vi "Toggle Selection.vi"(8 "error in (no error)":errorcluster, 10 "Tag":string, 11 "TreeSelectionHierarchal in":refnum<class "TreeSelectionHierarchal.lvclass">) -> (0 "error out":errorcluster, 3 "TreeSelectionHierarchal out":refnum<class "TreeSelectionHierarchal.lvclass">)   [LabVIEW 2015, in "TreeSelectionHierarchal.lvclass"]
doc: "<b> </b> <b> </b>\n©2016 Q Software Innovations, LLC (QSI)\nwritten by Quentin Alldredge\nproduced in LabVIEW 2015\n\nsupport@qsoftwareinnovations.com\nwww.qsoftwareinnovations.com\n\nAll rights reserved.\n\nRedistribution and use in source and binary forms, with or without modification, are permitted provided that the following conditions are met:\n\n * Redistributions of source code must retain the above copyright notice, this list of conditions and the following disclaimer.\n * Redistributions in binary form must reproduce the above copyright notice, this list of conditions and the following disclaimer in the documentation and/or other materials provided with the distribution.\n * Neither the name of Q Software Innovations, LLC. nor the names of its contributors may be used to endorse or promote products derived from this software without specific prior written permission.\n\nTHIS SOFTWARE IS PROVIDED BY THE COPYRIGHT HOLDERS AND CONTRIBUTORS \"AS IS\" AND ANY EXPRESS OR IMPLIED WARRANTIES, INCLUDING, BUT NOT LIMITED TO, THE IMPLIED WARRANTIES OF MERCHANTABILITY AND FITNESS FOR A PARTICULAR PURPOSE ARE DISCLAIMED. IN NO EVENT SHALL THE COPYRIGHT OWNER OR CONTRIBUTORS BE LIABLE FOR ANY DIRECT, INDIRECT, INCIDENTAL, SPECIAL, EXEMPLARY, OR CONSEQUENTIAL DAMAGES (INCLUDING, BUT NOT LIMITED TO, PROCUREMENT OF SUBSTITUTE GOODS OR SERVICES; LOSS OF USE, DATA, OR PROFITS; OR BUSINESS INTERRUPTION) HOWEVER CAUSED AND ON ANY THEORY OF LIABILITY, WHETHER IN CONTRACT, STRICT LIABILITY, OR TORT (INCLUDING NEGLIGENCE OR OTHERWISE) ARISING IN ANY WAY OUT OF THE USE OF THIS SOFTWARE, EVEN IF ADVISED OF THE POSSIBILITY OF SUCH DAMAGE."
uses:
  TreeSelectionHierarchal.lvclass
  TreeControl/TreeControl.lvclass
  TreeSelection/TreeSelection.lvclass
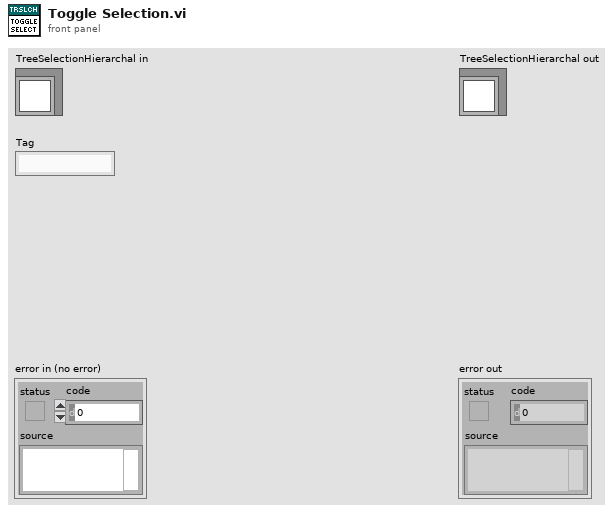
[diagram p1: front panel]
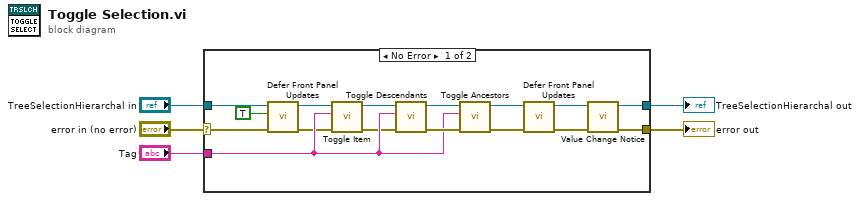
[diagram p0: block diagram]
diagram:
  n1 = case shown="No Error" "error in (no error)" {
    selector: "error in (no error)" -> [w20 w22]
    tunnel: "TreeSelectionHierarchal in" -> [w21 w23]
    tunnel: [w8 w23] -> w3
    tunnel: [w6 w22] -> w2
    tunnel: "Tag" -> [w12 _]
    frame No Error {
      n2 = call "Defer Front Panel Updates.vi"("error in (no error)"=w20, "Defer Panel Updates (F)"=TRUE, "Tree in"=w21) -> ("error out"=w11:errorcluster, "Tree (dup)"=w14:refnum<class "TreeSelectionHierarchal.lvclass">)  [unwired: 7 in]
      n3 = call "Toggle Item.vi"("error in (no error)"=w11, "Tag"=w12, "TreeSelection in"=w14) -> ("error out"=w10:errorcluster, "TreeSelection out"=w13:refnum<class "TreeSelectionHierarchal.lvclass">)  [unwired: 7 in]
      n4 = call "Toggle Descendants.vi"("error in (no error)"=w10, "Tag"=w12, "TreeHier in"=w13) -> ("error out"=w18:errorcluster, "TreeHier out"=w19:refnum<class "TreeSelectionHierarchal.lvclass">)  [unwired: 7 in]
      n5 = call "Toggle Ancestors.vi"("error in (no error)"=w18, "Tag"=w12, "TreeHier in"=w19) -> ("error out"=w15:errorcluster, "TreeHier out"=w16:refnum<class "TreeSelectionHierarchal.lvclass">)  [unwired: 7 in]
      n6 = call "Defer Front Panel Updates.vi"("error in (no error)"=w15, "Tree in"=w16) -> ("error out"=w7:errorcluster, "Tree (dup)"=w9:refnum<class "TreeSelectionHierarchal.lvclass">)  [unwired: 8 in]
      n7 = call "Value Change Notice.vi"("error in (no error)"=w7, "TreeSelection in"=w9) -> ("error out"=w6:errorcluster, "TreeSelection out"=w8:refnum<class "TreeSelectionHierarchal.lvclass">)  [unwired: 8 in]
    }
    frame Error {
    }
  }
  "error out" <- w2
  "TreeSelectionHierarchal out" <- w3
